vi "main.vi"() -> ()   [LabVIEW 2015]
uses:
  <vilib>/addons/database/Connection.llb/Conn ObjectReference.ctl
  <vilib>/Utility/miscctls.llb/LVPointTypeDef.ctl
  <vilib>/addons/database/Connection.llb/Conn Properties.ctl
  <vilib>/addons/database/Auxilliary.llb/DB Tools Transaction.ctl
  <vilib>/addons/database/Connection.llb/DB Tools Open Connec (Path).vi
  <vilib>/addons/database/Connection.llb/Conn Set Properties.vi
  <vilib>/addons/database/Connection.llb/Conn Transaction.vi
  <vilib>/addons/database/NI_Database_API.lvlib
panel:
  out "server":string
  out "THONG BAO":string
  in  "IP":string
  out "resulting string":string
  in  "Mo ta":string
  out "valid_program_name":string
  out "Note":string="Ten chuong trinh:\nKIEM KE\nCAT DAP\nBAN TU DONG\nPARTSET\nLINE CONVEYOR"
  in  "Ten chuong trinh":string
  out "valid_file":string
  out "valid_path_server":string
  in  "File chuong trinh":path
  in  "Note Error":string
  in  "Duong dan luu file":string="\\\\192.168.1.5\\data\\EN\\1. UPDATE"
  out "info":T1
  out "conn ref":T2
  in  "Stop Button":bool
  in  "upload":bool
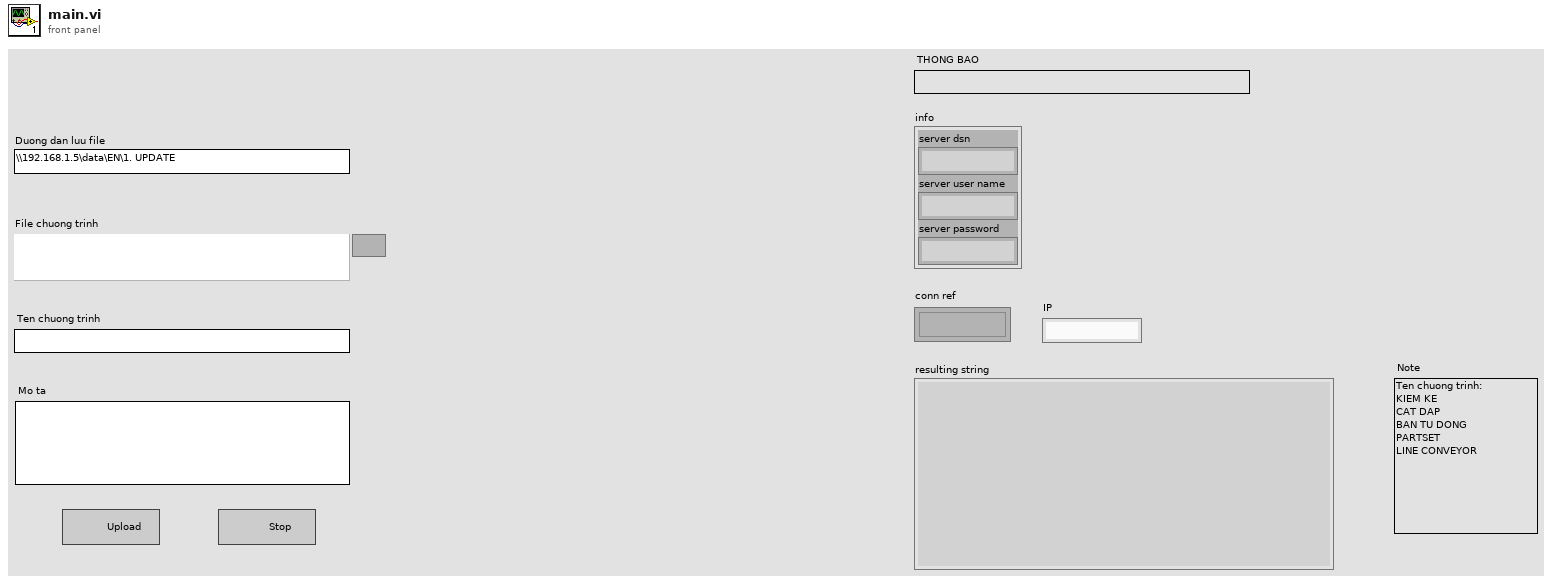
[diagram p1: front panel]
types:
  T1 = cluster{"server dsn":string, "server user name":string, "server password":string}
  T2 = typedef "NI_Database_API.lvlib/Conn ObjectReference.ctl" = refnum<k1>
  T3 = typedef "LVPointTypeDef.ctl" = cluster{"Horizontal":i16, "Vertical":i16}
  T4 = enum32{"invalid app kind", "Development System", "Run Time System", "Student Edition", "Embedded LabVIEW", "Evaluation", "Custom"}
  T5 = enum16{"open", "replace", "create", "open or create", "replace or create", "replace or create with confirmation"}
  T6 = typedef "NI_Database_API.lvlib/Conn Properties.ctl" = cluster{"command timeout (s)":i32, "connection string":string, "default database":string, "provider":string}
  T7 = typedef "NI_Database_API.lvlib/DB Tools Transaction.ctl" = enum16{"begin", "commit", "rollback"}
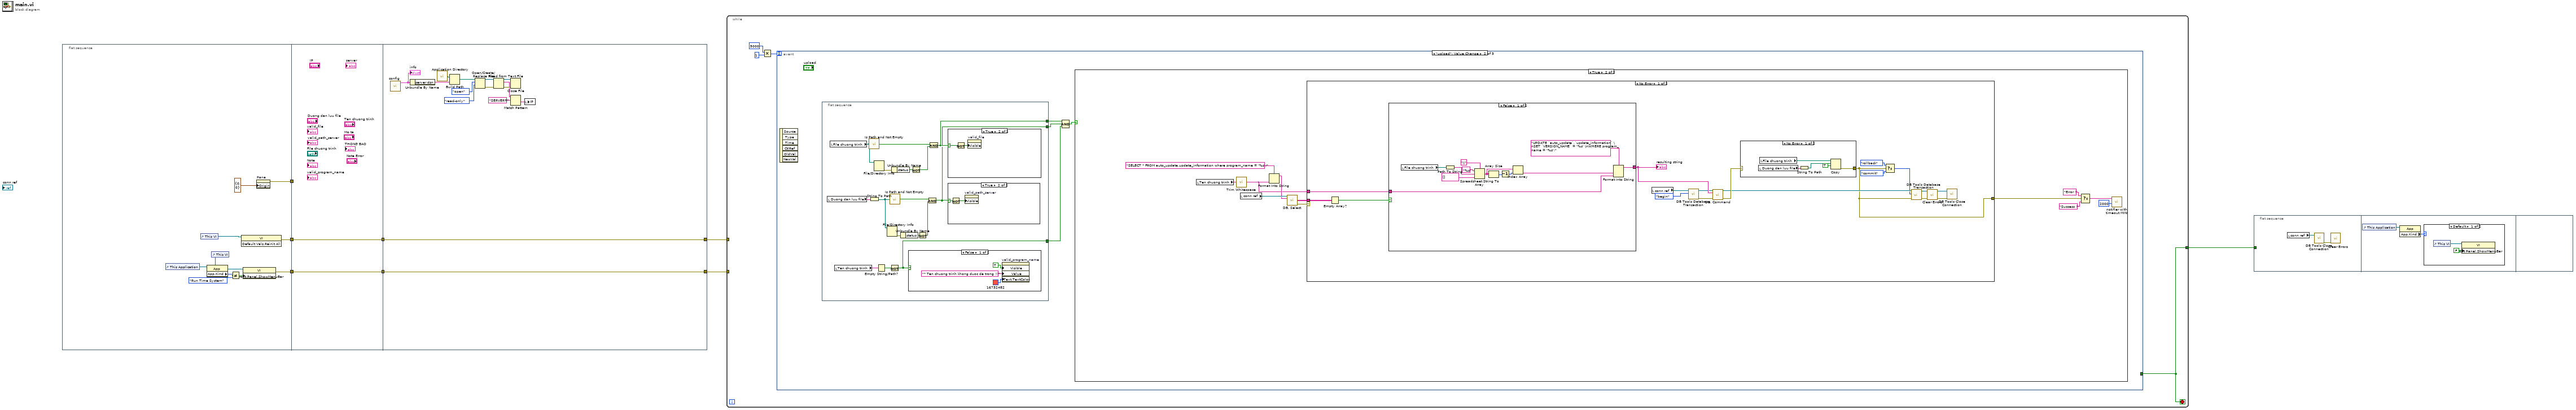
[diagram p0: block diagram]
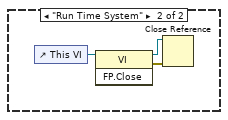
[diagram p2: hidden frame]
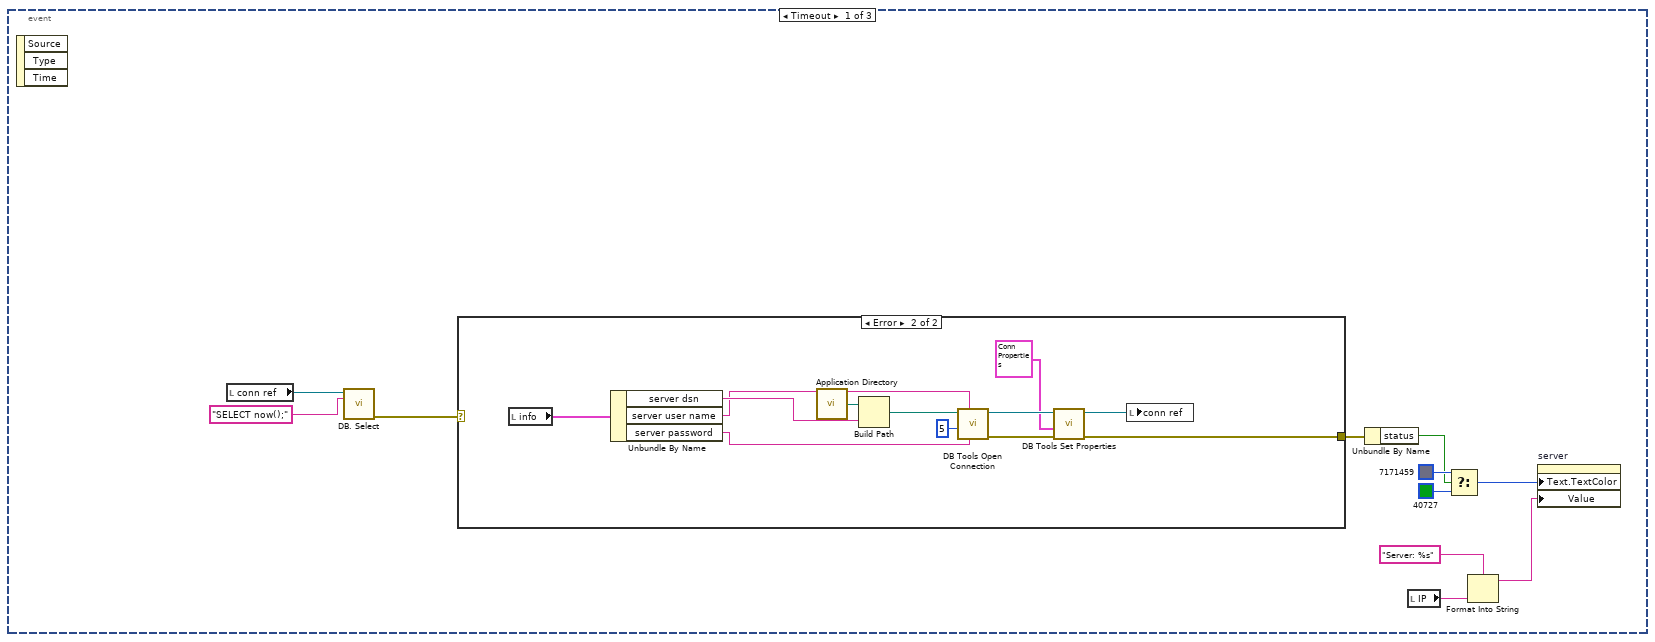
[diagram p3: hidden frame]
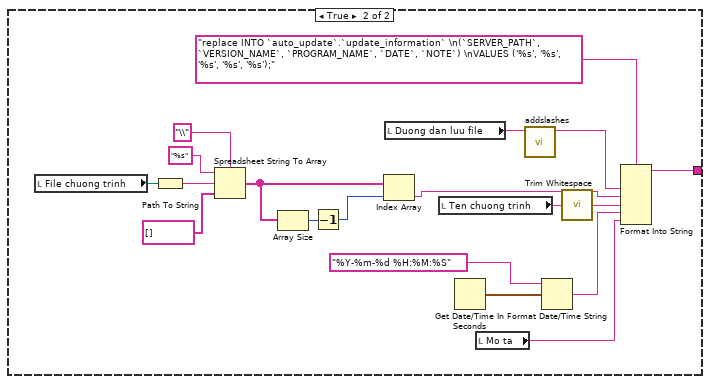
[diagram p7: hidden frame]
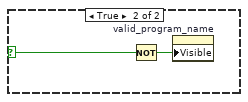
[diagram p9: hidden frame]
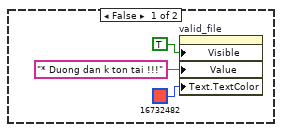
[diagram p10: hidden frame]
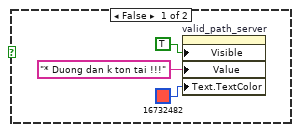
[diagram p11: hidden frame]
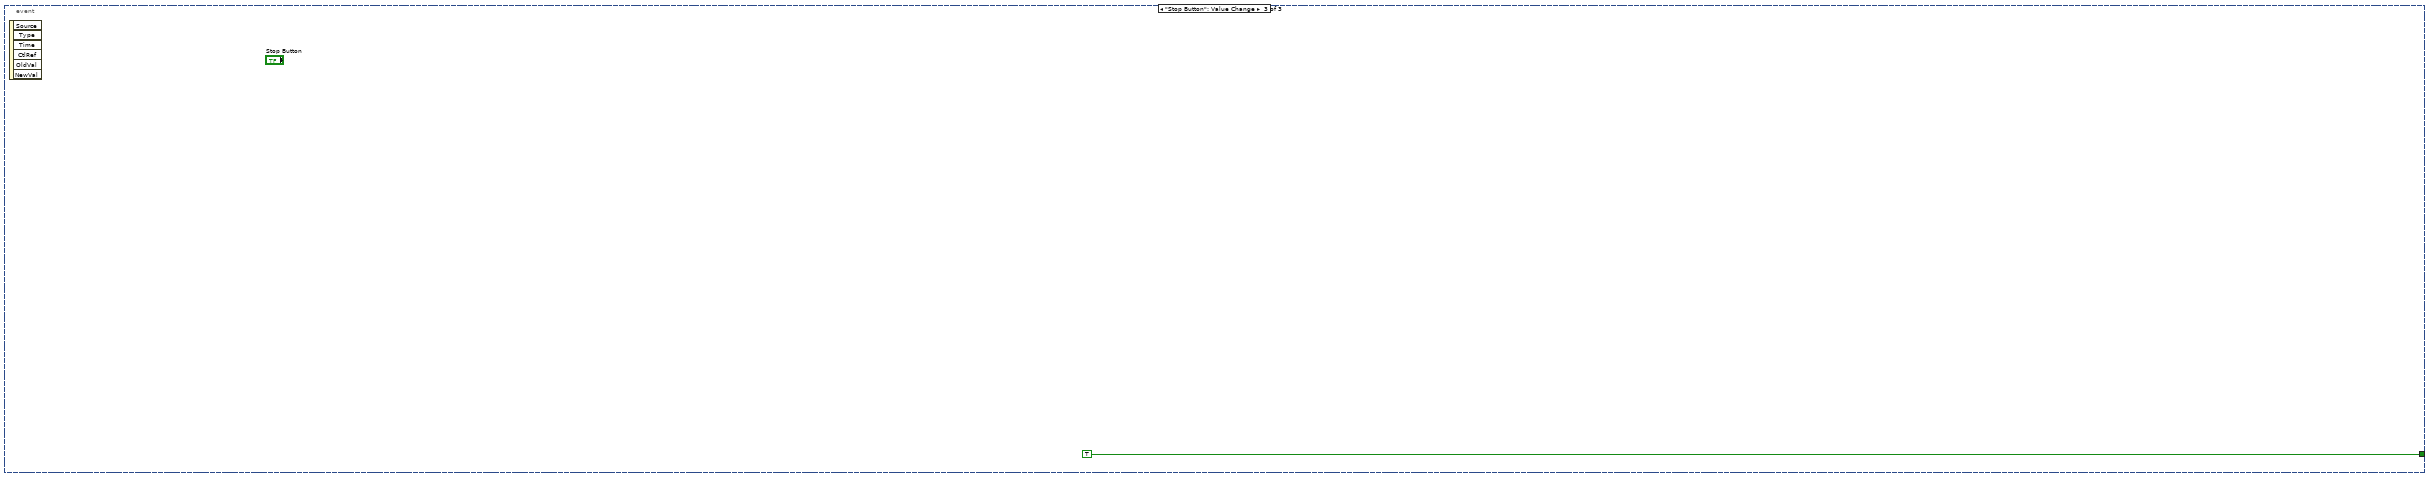
[diagram p12: hidden frame]
diagram:
  n1 = flat-sequence {
    tunnel: [w12] -> w5
    tunnel: [w11] -> w3
    tunnel: [w9] -> w1
    tunnel: w5 -> [w20]
    tunnel: [w20] -> w4
    tunnel: w3 -> [w19]
    tunnel: [w19] -> w2
    tunnel: w1 -> [_]
    tunnel: [w34] -> w7
    tunnel: [w35] -> w8
    tunnel: w4 -> [w35]
    tunnel: w2 -> [w34]
    frame #0 {
      n2 = control-ref of="This Application"() -> (w13:refnum<vi>)
      n3 = control-ref of="This VI"() -> (w18:refnum<vi>)
      n4 = property class="App"(reference=w13) -> ("App.Kind"=w14:T4)  [unwired: 1 in, 2 out]
      n5 = control-ref of="This VI"() -> (w16:refnum<vi>)
      n6 = Not Equal?(x=w14, y=T4."Run Time System") -> (x != y?=w17:bool)
      n7 = invoke class="VI" method="Default Vals.Reinit All"(reference=w18) -> (error out=w11:errorcluster)  [unwired: 2 in, 2 out]
      n8 = property class="VI"(reference=w16, "Front Panel.ShowMenuBar"=w17) -> (error out=w12:errorcluster)  [unwired: 1 in, 1 out]
      n9 = property on="Pane" class="Pane"("Origin"=T3 {"Horizontal"=0, "Vertical"=0}) -> (error out=w9:errorcluster)  [unwired: 2 in, 1 out]
    }
    frame #1 {
    }
    frame #2 {
      n10 = call "config.vi"() -> ("info"=w33:T1)  [unwired: 11 in]
      "info" <- w33
      n11 = Unbundle By Name(w33) -> ("server dsn"=w32:string)
      n12 = call <vilib>:"Application Directory.vi"() -> ("Application Directory"=w31:path)
      n13 = Build Path(base path=w31, name or relative path=w32) -> (appended path=w30:path)
      n14 = Open/Create/Replace File(file path (use dialog)=w30, operation (0:open)=T5."open", access (0:read/write)=enum16{"read/write", "read-only", "write-only"}."read-only") -> (refnum out=w26:refnum<file>, error out=w27:errorcluster)  [unwired: 3 in, 1 out]
      n15 = Read from Text File(file (use dialog)=w26, error in=w27) -> (refnum out=w25:refnum<file>, text=w23:string, error out=w24:errorcluster)  [unwired: 2 in, 1 out]
      n16 = Close File(refnum=w25, error in=w24) -> ()  [unwired: 2 out]
      n17 = Match Pattern(string=w23, regular expression="SERVER=") -> (after substring=w21:string)  [unwired: 1 in, 3 out]
      n18 = local write "IP"(w21) -> ()
    }
  }
  n19 = while {
    tunnel: w8 -> [_]
    tunnel: w7 -> [_]
    tunnel: [w39] -> w6
    stop <- w39 stop-if-true
    n20 = Multiply(x=5000, y=1) -> (x*y=w36:i32)
    n21 = event shown="[1] \"upload\": Value Change" {
      selector: _ -> [_ _ _]
      dyn-events: _ -> [_ _ _]
      timeout: w36 -> [_ _ _]
      tunnel: [_ _ TRUE] -> w39
      event Timeout {
        n22 = event-data() -> ()  [unwired: 1 in, 3 out]
        n23 = local read "conn ref"() -> (w50:T2)
        n24 = call "DB. Select.vi"("conn ref"=w50, "SQL query"="SELECT now();") -> ("error out"=w48:errorcluster)  [unwired: 9 in, 4 out]
        n25 = case shown="Error" w48 {
          tunnel: [_ w51] -> w47
          frame No Error {
          }
          frame Error {
            n26 = local read "info"() -> (w62:T1)
            n27 = Unbundle By Name(w62) -> ("server dsn"=w60:string, "server user name"=w58:string, "server password"=w57:string)
            n28 = call <vilib>:"Application Directory.vi"() -> ("Application Directory"=w61:path)
            n29 = Build Path(base path=w61, name or relative path=w60) -> (appended path=w59:path)
            n30 = call-poly <vilib>:"DB Tools Open Connection.vi"("password"=w57, "userID"=w58, "connection timeout (15)"=5, "connection information"=w59) -> ("error out"=w54:errorcluster, "connection reference"=w55:T2)  [unwired: 4 in]
            n31 = call-poly <vilib>:"DB Tools Set Properties.vi"("error in (no error)"=w54, "connection properties"=T6 {"command timeout (s)"=15, "connection string"="", "default database"="asti_wh_management", "provider"=""}, "connection reference"=w55) -> ("error out"=w51:errorcluster, "connection reference out"=w52:T2)  [unwired: 3 in]
            n32 = local write "conn ref"(w52) -> ()
          }
        }
        n33 = Unbundle By Name(w47) -> ("status"=w44:bool)
        n34 = local read "IP"() -> (w41:string)
        n35 = Select(t=u32 7171459, s=w44, f=u32 40727) -> (s? t:f=w43:u32)
        n36 = Format Into String(format string="Server: %s", w41) -> (resulting string=w40:string)  [unwired: 2 in, 1 out]
        n37 = property on="server" class="Str"("Text.TextColor"=w43, "Value"=w40) -> ()  [unwired: 2 in, 2 out]
      }
      event "upload": Value Change {
        n38 = event-data() -> ()  [unwired: 1 in, 6 out]
        n39 = flat-sequence {
          tunnel: [w139] -> w66
          tunnel: [w138] -> w65
          tunnel: [w135] -> w63
          frame #0 {
            n40 = local read "Duong dan luu file"() -> (w149:string)
            n41 = local read "File chuong trinh"() -> (w147:path)
            n42 = local read "Ten chuong trinh"() -> (w137:string)
            n43 = call <vilib>:"Is Path and Not Empty.vi"("path"=w147) -> ("Is Path and Not Empty?"=w141:bool)  [unwired: 4 in]
            n44 = String To Path(string=w149) -> (path=w148:path)
            n45 = File/Directory Info(path=w147) -> (error out=w146:errorcluster)  [unwired: 1 in, 6 out]
            n46 = Empty String/Path?(string/path=w137) -> (empty?=w136:bool)
            n47 = File/Directory Info(path=w148) -> (error out=w145:errorcluster)  [unwired: 1 in, 6 out]
            n48 = call <vilib>:"Is Path and Not Empty.vi"("path"=w148) -> ("Is Path and Not Empty?"=w143:bool)  [unwired: 4 in]
            n49 = Not(x=w136) -> (.not. x?=w135:bool)
            n50 = Unbundle By Name(w146) -> ("status"=w140:bool)
            n51 = Unbundle By Name(w145) -> ("status"=w144:bool)
            n52 = case shown="False" w135 {
              selector: w135 -> [_ w154]
              frame False {
                n53 = property on="valid_program_name" class="Str"("Visible"=TRUE, "Value"="* Ten chuong trinh khong duoc de trong !!!" ("valid_path_server"), "Text.TextColor"=u32 16732482) -> ()  [unwired: 2 in, 2 out]
              }
              frame True {
                n54 = Not(x=w154) -> (.not. x?=w153:bool)
                n55 = property on="valid_program_name" class="Str"("Visible"=w153) -> ()  [unwired: 2 in, 2 out]
              }
            }
            n56 = Not(x=w140) -> (.not. x?=w134:bool)
            n57 = Not(x=w144) -> (.not. x?=w142:bool)
            n58 = And(x=w143, y=w142) -> (x .and. y?=w138:bool)
            n59 = And(x=w141, y=w134) -> (x .and. y?=w139:bool)
            n60 = case shown="True" w139 {
              selector: w139 -> [_ w158]
              frame False {
                n61 = property on="valid_file" class="Str"("Visible"=TRUE, "Value"="* Duong dan k ton tai !!!" ("valid_path_server"), "Text.TextColor"=u32 16732482) -> ()  [unwired: 2 in, 2 out]
              }
              frame True {
                n62 = Not(x=w158) -> (.not. x?=w159:bool)
                n63 = property on="valid_file" class="Str"("Visible"=w159) -> ()  [unwired: 2 in, 2 out]
              }
            }
            n64 = case shown="True" w138 {
              selector: w138 -> [_ w164]
              frame False {
                n65 = property on="valid_path_server" class="Str"("Visible"=TRUE, "Value"="* Duong dan k ton tai !!!" ("valid_path_server"), "Text.TextColor"=u32 16732482) -> ()  [unwired: 2 in, 2 out]
              }
              frame True {
                n66 = Not(x=w164) -> (.not. x?=w163:bool)
                n67 = property on="valid_path_server" class="Str"("Visible"=w163) -> ()  [unwired: 2 in, 2 out]
              }
            }
          }
        }
        n68 = Compound Arithmetic op=AND(w66, w65, w63) -> (w64:bool)
        n69 = case shown="True" w64 {
          frame False {
          }
          frame True {
            n70 = local read "Ten chuong trinh"() -> (w76:string)
            n71 = call <vilib>:"Trim Whitespace.vi"("string"=w76) -> ("trimmed string"=w67:string)  [unwired: 1 in]
            n72 = local read "conn ref"() -> (w78:T2)
            n73 = Format Into String(format string="SELECT * FROM auto_update.update_information where program_name = '%s';" ("SQL query"), w67) -> (resulting string=w75:string)  [unwired: 2 in, 1 out]
            n74 = call "DB. Select.vi"("conn ref"=w78, "SQL query"=w75) -> ("data"=w68:string[][], "error out"=w74:errorcluster)  [unwired: 9 in, 3 out]
            n75 = case shown="No Error" w74 {
              selector: w74 -> [_ w133]
              tunnel: [w79 w133] -> w69
              tunnel: w68 -> [w95 _]
              tunnel: w67 -> [w92 _]
              frame No Error {
                n76 = Empty Array?(array=w95) -> (empty?=w93:bool)
                n77 = case shown="False" w93 {
                  tunnel: [w112 w116] -> w94
                  tunnel: w92 -> [w111 _]
                  frame False {
                    n78 = local read "File chuong trinh"() -> (w110:path)
                    n79 = Path To String(path=w110) -> (string=w109:string)
                    n80 = Spreadsheet String To Array(delimiter (Tab)="\\", format string="%s", spreadsheet string=w109, array type (2D Dbl)=string[] []) -> (array=w103:string[])
                    n81 = Array Size(array=w103) -> (size(s)=w105:i32)
                    n82 = Decrement(x=w105) -> (x-1=w104:i32)
                    n83 = Index Array(array=w103, index=w104) -> (element=w102:string)
                    n84 = Format Into String(format string="UPDATE `auto_update`.`update_information` \nSET `VERSION_NAME` = '%s' \nWHERE program_name = '%s';", w102, w111) -> (resulting string=w112:string)  [unwired: 2 in, 1 out]
                  }
                  frame True {
                    n85 = local read "File chuong trinh"() -> (w132:path)
                    n86 = Path To String(path=w132) -> (string=w131:string)
                    n87 = Spreadsheet String To Array(delimiter (Tab)="\\" ("format string"), format string="%s", spreadsheet string=w131, array type (2D Dbl)=string[] []) -> (array=w127:string[])
                    n88 = Array Size(array=w127) -> (size(s)=w126:i32)
                    n89 = Decrement(x=w126) -> (x-1=w125:i32)
                    n90 = Index Array(array=w127, index=w125) -> (element=w123:string)
                    n91 = local read "Duong dan luu file"() -> (w115:string)
                    n92 = local read "Ten chuong trinh"() -> (w122:string)
                    n93 = Get Date/Time In Seconds() -> (seconds since 1Jan1904=w119:timestamp)
                    n94 = local read "Mo ta"() -> (w120:string)
                    n95 = call "addslashes.vi"("input string"=w115) -> ("addslashes"=w114:string)  [unwired: 10 in]
                    n96 = Format Date/Time String(time format string (%c)="%Y-%m-%d %H:%M:%S" ("format string"), seconds (now)=w119) -> (date/time string=w117:string)  [unwired: 1 in]
                    n97 = call <vilib>:"Trim Whitespace.vi"("string"=w122) -> ("trimmed string"=w121:string)  [unwired: 1 in]
                    n98 = Format Into String(format string="replace INTO `auto_update`.`update_information` \n(`SERVER_PATH`, `VERSION_NAME`, `PROGRAM_NAME`, `DATE`, `NOTE`) \nVALUES ('%s', '%s', '%s', '%s', '%s');", w114, w123, w121, w117, w120) -> (resulting string=w116:string)  [unwired: 2 in, 1 out]
                  }
                }
                "resulting string" <- w94
                n99 = local read "conn ref"() -> (w91:T2)
                n100 = call-poly <vilib>:"DB Tools Database Transaction.vi"("operation (begin)"=DB_Tools_Transaction."begin", "connection reference"=w91) -> ("error out"=w88:errorcluster, "connection reference out"=w90:T2)  [unwired: 4 in]
                n101 = call "DB. Command.vi"("conn ref"=w90, "SQL query"=w94, "error in (no error)"=w88) -> ("conn ref 2"=w86:T2, "error out"=w87:errorcluster)  [unwired: 11 in]
                n102 = case shown="No Error" w87 {
                  selector: w87 -> [_ w101]
                  tunnel: [w96 w101] -> w79
                  frame No Error {
                    n103 = local read "Duong dan luu file"() -> (w99:string)
                    n104 = local read "File chuong trinh"() -> (w100:path)
                    n105 = String To Path(string=w99) -> (path=w98:path)
                    n106 = Copy(9:TRUE ("overwrite (F)"), 10:w98, 11:w100) -> (0:w96:errorcluster)  [unwired: 2 in, 2 out]
                  }
                  frame Error {
                  }
                }
                n107 = Select(t=DB_Tools_Transaction."rollback" ("operation (begin)"), s=w79, f=DB_Tools_Transaction."commit" ("operation (begin)")) -> (s? t:f=w83:T7)
                n108 = call-poly <vilib>:"DB Tools Database Transaction.vi"("error in (no error)"=w79, "operation (begin)"=w83, "connection reference"=w86) -> ("error out"=w82:errorcluster, "connection reference out"=w81:T2)  [unwired: 3 in]
                n109 = call <vilib>:"Clear Errors.vi"("error in (no error)"=w82) -> ("error out"=w80:errorcluster)  [unwired: 5 in, 1 out]
                n110 = call <vilib>:"DB Tools Close Connection.vi"("error in (no error)"=w80, "connection reference"=w81) -> ()  [unwired: 5 in, 1 out]
              }
              frame Error {
              }
            }
            n111 = Select(t="Error !", s=w69, f="Success !") -> (s? t:f=w73:string)
            n112 = call "notifier with timeout MINI.vi"("milliseconds to wait"=u32 2000, "message"=w73) -> ()  [unwired: 8 in, 2 out]
          }
        }
      }
      event "Stop Button": Value Change {
        n113 = event-data() -> ()  [unwired: 1 in, 6 out]
      }
    }
  }
  n114 = flat-sequence {
    tunnel: w6 -> [_]
    frame #0 {
      n115 = local read "conn ref"() -> (w167:T2)
      n116 = call <vilib>:"DB Tools Close Connection.vi"("connection reference"=w167) -> ("error out"=w166:errorcluster)  [unwired: 6 in]
      n117 = call <vilib>:"Clear Errors.vi"("error in (no error)"=w166) -> ()  [unwired: 5 in, 2 out]
    }
    frame #1 {
      n118 = control-ref of="This Application"() -> (w168:refnum<vi>)
      n119 = property class="App"(reference=w168) -> ("App.Kind"=w169:T4)  [unwired: 1 in, 2 out]
      n120 = case shown="Default" w169 {
        frame Default {
          n121 = control-ref of="This VI"() -> (w171:refnum<vi>)
          n122 = property class="VI"(reference=w171, "Front Panel.ShowMenuBar"=FALSE ("Front Panel Window:Show Menu Bar")) -> ()  [unwired: 1 in, 2 out]
        }
        frame "Run Time System" {
          n123 = control-ref of="This VI"() -> (w174:refnum<vi>)
          n124 = invoke class="VI" method="FP.Close"(reference=w174) -> (reference out=w172:refnum<vi>, error out=w173:errorcluster)  [unwired: 2 in, 1 out]
          n125 = Close Reference(reference=w172, error in (no error)=w173) -> ()  [unwired: 1 out]
        }
      }
    }
    frame #2 {
    }
  }
